vi "Center.vi"(1 "Power":dbl, 2 "Rev":bool, 3 "Fwd":bool) -> (0 "Center Power":dbl)   [LabVIEW 2013]
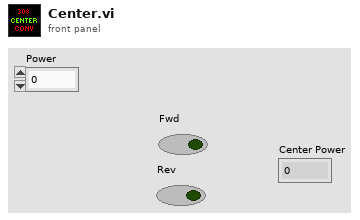
[diagram p1: front panel]
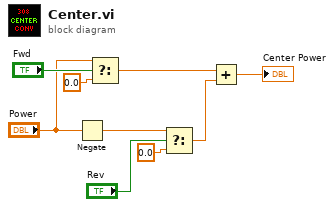
[diagram p0: block diagram]
diagram:
  n1 = Negate(x="Power") -> (-x=w5:dbl)
  n2 = Select(t="Power", s="Fwd", f=0.0) -> (s? t:f=w2:dbl)
  n3 = Select(t=w5, s="Rev", f=0.0) -> (s? t:f=w3:dbl)
  n4 = Add(x=w2, y=w3) -> (x+y=→"Center Power":dbl)
